vi "Get Measurement Details.vi"(8 "error in":errorcluster) -> (0 "error out":errorcluster, 1 "measurement annotations":T1[](array[typedef]), 2 "service class":string, 3 "measurement details":T2)   [LabVIEW 2021, in "Table and Multicolumn Listbox.lvlib"]
uses:
  Table and Multicolumn Listbox.lvlib
  <vilib>/MeasurementLink/MeasurementLink Measurement Server/Helpers/TypeDefs/Measurement Details.ctl
  <vilib>/MeasurementLink/MeasurementLink Measurement Server/Helpers/TypeDefs/Measurement Annotation.ctl
  <vilib>/MeasurementLink/MeasurementLink Measurement Server/MeasurementLink Measurement Server.lvlib
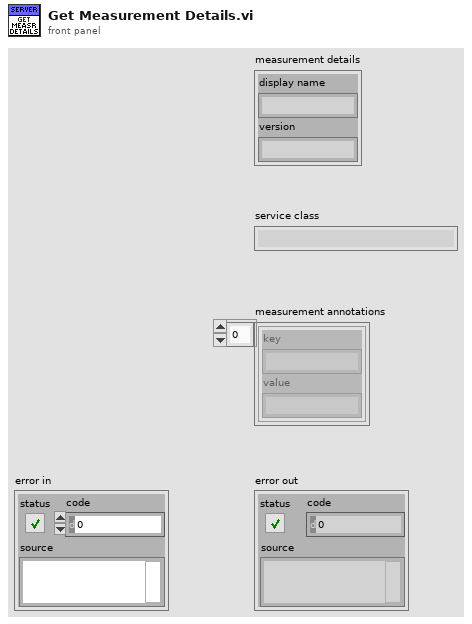
[diagram p1: front panel]
types:
  T1 = typedef "MeasurementLink Measurement Server.lvlib/Measurement Annotation.ctl" = cluster{"key":string, "value":string}
  T2 = typedef "MeasurementLink Measurement Server.lvlib/Measurement Details.ctl" = cluster{"display name":string, "version":string}
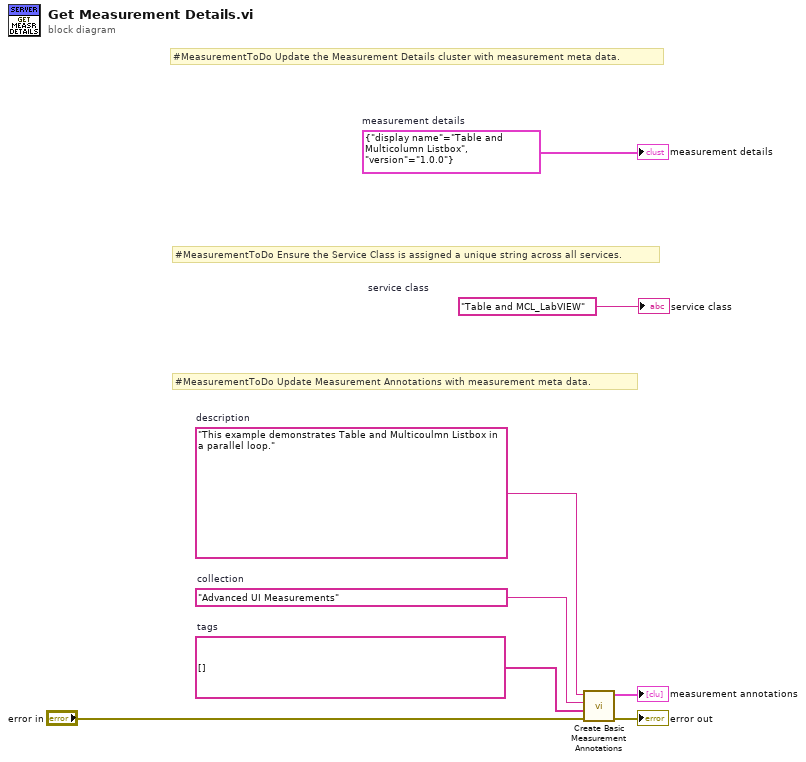
[diagram p0: block diagram]
diagram:
  w1 = string[] []  # tags
  w2 = "Advanced UI Measurements"  # collection
  w3 = "This example demonstrates Table and Multicoulmn Listbox in a parallel loop."  # description
  w7 = T2 {"display name"="Table and Multicolumn Listbox", "version"="1.0.0"}  # measurement details
  w8 = "Table and MCL_LabVIEW"  # service class
  # "#MeasurementToDo Update Measurement Annotations with measurement meta data."
  # "#MeasurementToDo Ensure the Service Class is assigned a unique string across all services."
  # "#MeasurementToDo Update the Measurement Details cluster with measurement meta data."
  n1 = call <vilib>:"Create Basic Measurement Annotations.vi"("error in"="error in", "tags"=w1, "collection"=w2, "description"=w3) -> ("error out"=→"error out":errorcluster, "measurement annotations"=→"measurement annotations":T1[])  [unwired: 6 in]
  "measurement details" <- w7
  "service class" <- w8
